vi "Pre Launch Init.vi"(11 "SpectrumAnalyzerUI in":refnum<class "SpectrumAnalyzerUI.lvclass">) -> (0 "error out":errorcluster, 3 "SpectrumAnalyzerUI out":refnum<class "SpectrumAnalyzerUI.lvclass">)   [LabVIEW 2023, in "SpectrumAnalyzerUI.lvlib" / "SpectrumAnalyzerUI.lvclass"]
doc: "(<B>Filename</B>: Actor Framework.lvlib:Actor.lvclass:Pre Launch Init.vi)\n\nDefines behavior that occurs after the Launch Nested Actor method is invoked but before the actor's Actor Core method begins running.\n\nBy default, this method does nothing. A descendant class may override it to define behavior."
uses:
  SpectrumAnalyzerUI.lvclass
  SpectrumAnalyzerUI.lvclass/SpectrumAnalyzerUI.ctl
  <vilib>/ActorFramework/Actor/Actor.lvclass
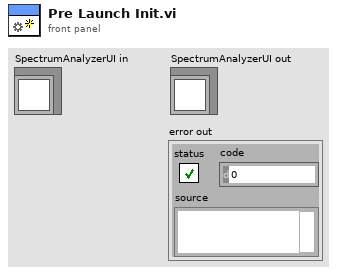
[diagram p1: front panel]
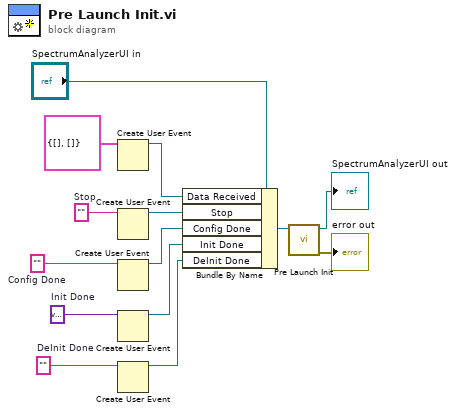
[diagram p0: block diagram]
diagram:
  w2 = variant  # Init Done
  w7 = ""  # DeInit Done
  w8 = ""  # Config Done
  w11 = ""  # Stop
  n1 = Create User Event(user event datatype=cluster{"Frequency":dbl[], "Amplitude":dbl[]} {"Frequency"=[], "Amplitude"=[]} ("Spectrum")) -> (user event=w3:refnum<user-event>)  [unwired: 1 in, 1 out]
  n2 = Create User Event(user event datatype=w11) -> (user event=w10:refnum<user-event>)  [unwired: 1 in, 1 out]
  n3 = Create User Event(user event datatype=w8) -> (user event=w9:refnum<user-event>)  [unwired: 1 in, 1 out]
  n4 = Create User Event(user event datatype=w2) -> (user event=w1:refnum<user-event>)  [unwired: 1 in, 1 out]
  n5 = Create User Event(user event datatype=w7) -> (user event=w6:refnum<user-event>)  [unwired: 1 in, 1 out]
  n6 = Bundle By Name(cluster="SpectrumAnalyzerUI in", "Data Received"=w3, "Stop"=w10, "Config Done"=w9, "Init Done"=w1, "DeInit Done"=w6) -> (w4:refnum<class "SpectrumAnalyzerUI.lvclass">)
  n7 = call-parent "Pre Launch Init.vi"("Actor in"=w4) -> ("error out"=→"error out":errorcluster, "Actor out"=→"SpectrumAnalyzerUI out":refnum<class "SpectrumAnalyzerUI.lvclass">)  [unwired: 9 in]
